vi "Acquire Measurement.vi"(8 "error in (no error)":errorcluster {"code" format="%.0x"}, 11 "VISA resource name":refnum<visa-resource-name>) -> (0 "error out":errorcluster {"code" format="%.0x"}, 2 "Trace Data":dbl[](array[numeric]) format="%^.3e", 3 "VISA resource name out":refnum<visa-resource-name>)   [LabVIEW 2015]
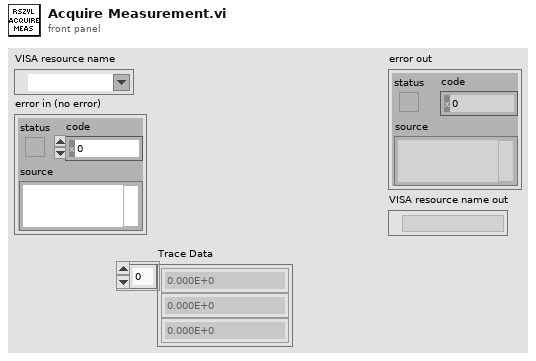
[diagram p1: front panel]
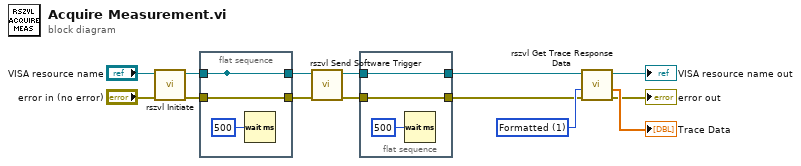
[diagram p0: block diagram]
diagram:
  w13 = 1 items=["Unformatted", "Formatted", "Unformatted With Trace Mathematics"] ("Data Format (Unformatted)")
  n1 = call <instrlib>:"rszvl Initiate.vi"("error in (no error)"="error in (no error)", "VISA resource name"="VISA resource name") -> ("error out"=w4:errorcluster, "VISA resource name out"=w3:refnum<visa-resource-name>)  [unwired: 8 in]
  n2 = flat-sequence {
    tunnel: [w15] -> _
    tunnel: w3 -> [w15]
    tunnel: [w17] -> w1
    tunnel: w4 -> [w17]
    tunnel: [w15] -> w2
    frame #0 {
      n3 = Wait (ms)(milliseconds to wait=u32 500) -> ()  [unwired: 1 out]
    }
  }
  n4 = call <instrlib>:"rszvl Send Software Trigger.vi"("error in (no error)"=w1, "VISA resource name"=w2) -> ("error out"=w6:errorcluster, "VISA resource name out"=w5:refnum<visa-resource-name>)  [unwired: 8 in]
  n5 = flat-sequence {
    tunnel: [w20] -> w12
    tunnel: w5 -> [w20]
    tunnel: [w19] -> w11
    tunnel: w6 -> [w19]
    frame #0 {
      n6 = Wait (ms)(milliseconds to wait=u32 500) -> ()  [unwired: 1 out]
    }
  }
  n7 = call <instrlib>:"rszvl Get Trace Response Data.vi"("error in (no error)"=w11, "Data Format (Unformatted)"=w13, "VISA resource name"=w12) -> ("error out"=→"error out":errorcluster, "Trace Data"=→"Trace Data":dbl[], "VISA resource name out"=→"VISA resource name out":refnum<visa-resource-name>)  [unwired: 6 in]
